vi "Motor Controller.vi"(6 "error in (no error)":errorcluster, 9 "Message Queues in":T1) -> (0 "error out":errorcluster)   [LabVIEW 2024]
uses:
  support/Message Queue/All Message Queues.ctl
  support/Message Queue/Message Cluster.ctl
  support/MotorBoolControlsIndicators.ctl
  support/MotorBoolControls.ctl
  support/MotorSpeedControls.ctl
  support/Message Queue/Enqueue Message (Single).vi
  <vilib>/addons/control/pid/pid.llb/PID (DBL).vi
  support/Message Queue/Message Queue.lvlib
  <vilib>/addons/control/pid/NI_PID_pid.lvlib
panel:
  out "Torque Measurement":dbl
  out "Setpoint Torque":dbl
  out "Setpoint Speed 2":dbl
  out "Setpoint Speed 1":dbl
  out "Sync":bool
  out "Async":bool
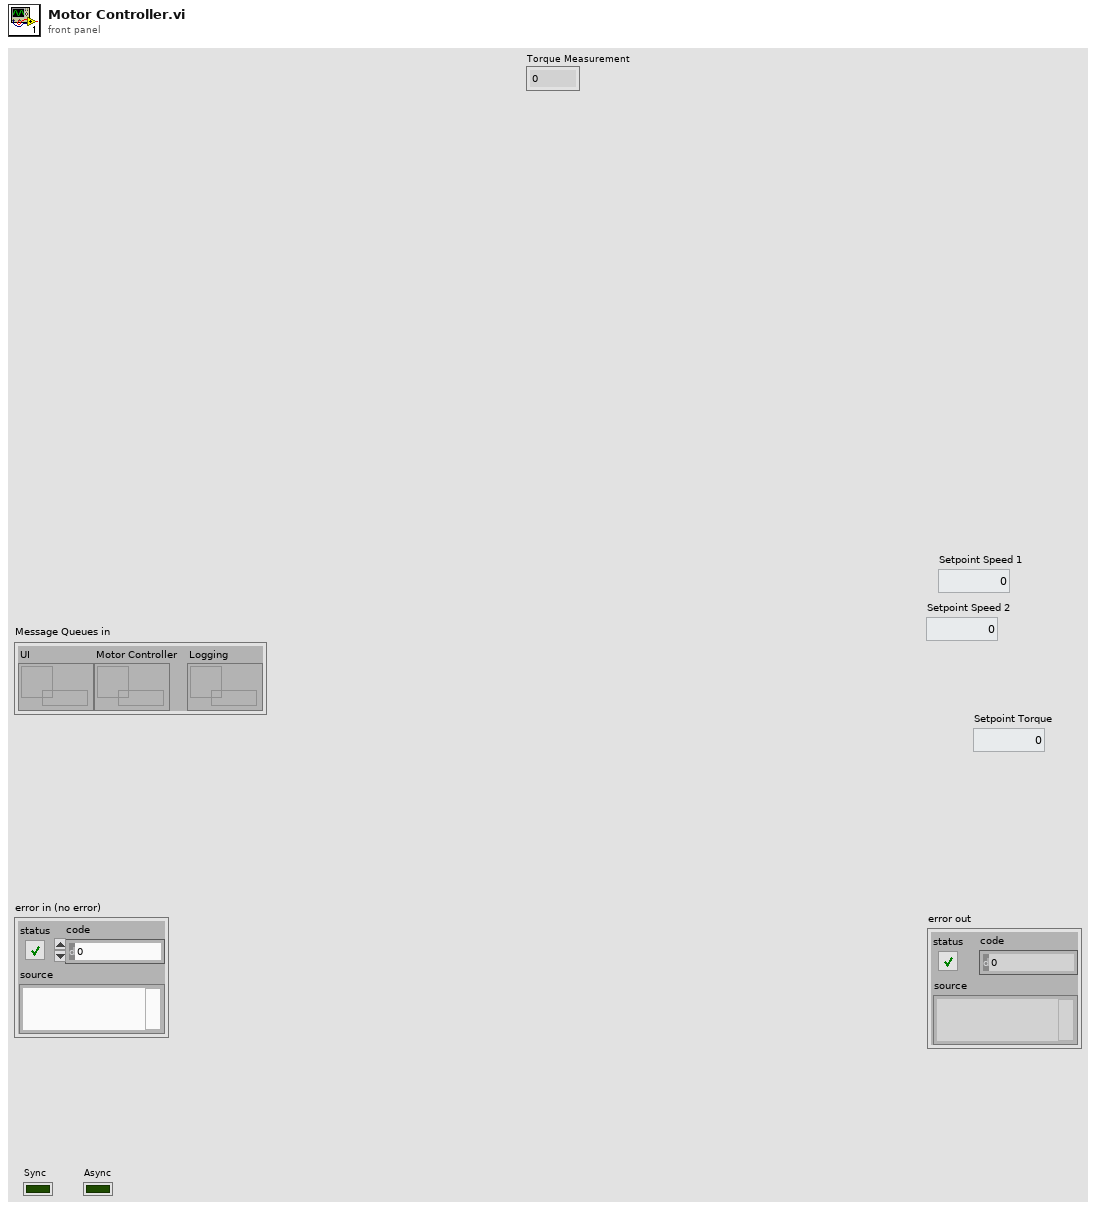
[diagram p1: front panel]
types:
  T1 = typedef "Message Queue.lvlib/All Message Queues.ctl" = cluster{"UI":refnum<queue>, "Motor Controller":refnum<queue>, "Logging":refnum<queue>}
  T2 = typedef "MotorBoolControlsIndicators.ctl" = cluster{"Motor 1 On":bool, "Motor 2 On":bool, "Motors Off":bool, "Start Motor 1 ":bool, "Start Motor 2":bool}
  T3 = typedef "MotorBoolControls.ctl" = cluster{"Motor1On":bool, "Motor2On":bool, "MotorsOff":bool, "StartMotor1":bool, "StartMotor2":bool}
  T4 = typedef "MotorSpeedControls.ctl" = cluster{"SetSpeed1":dbl, "SetSpeed 2":dbl}
  T5 = typedef "MotorStatusIndicators.ctl" = cluster{"Motor 1 Ok":bool, "Motor 2 ok":bool}
  T6 = typedef "ReadSpeed.ctl" = cluster{"SetSpeed1":dbl, "SetSpeed2":dbl, "ReadSpeed1":dbl, "ReadSpeed2":dbl}
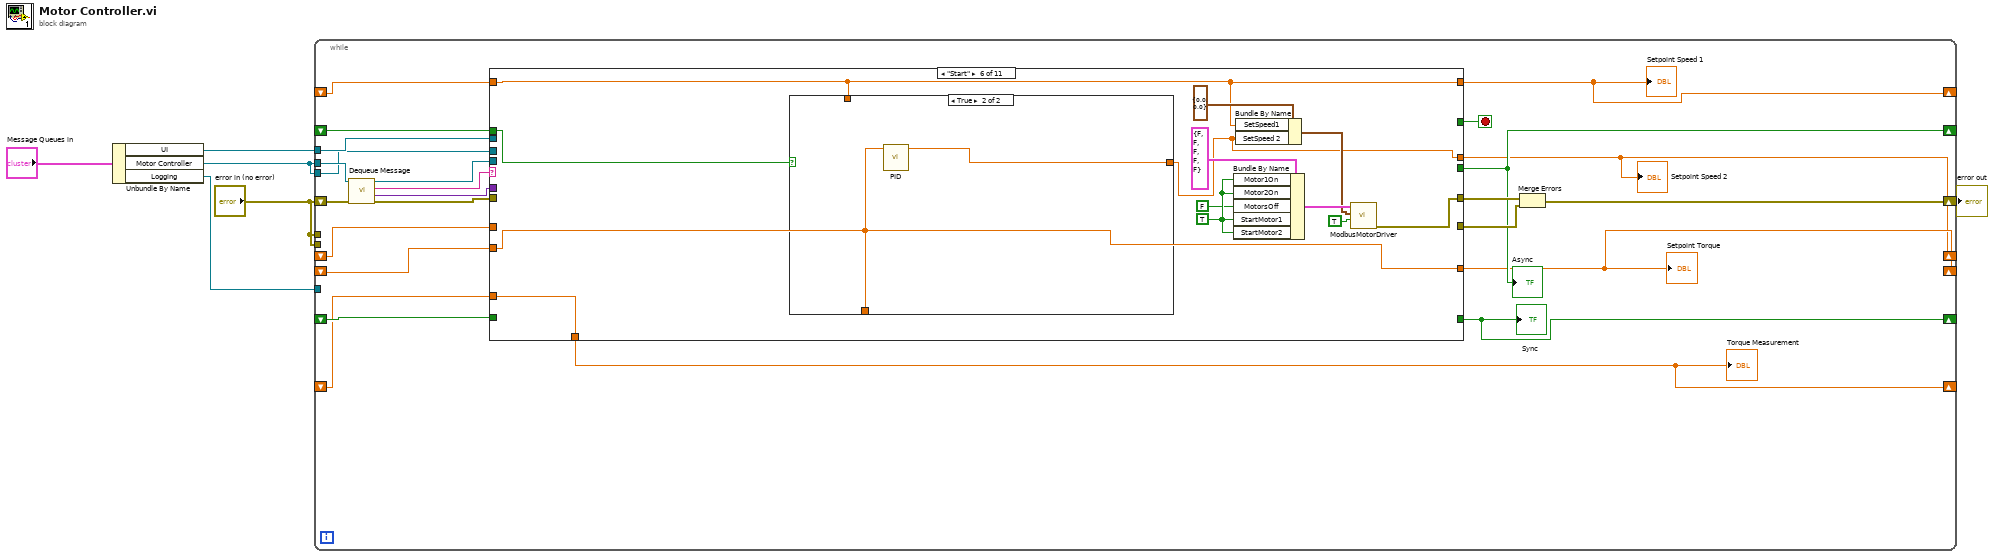
[diagram p0: block diagram]
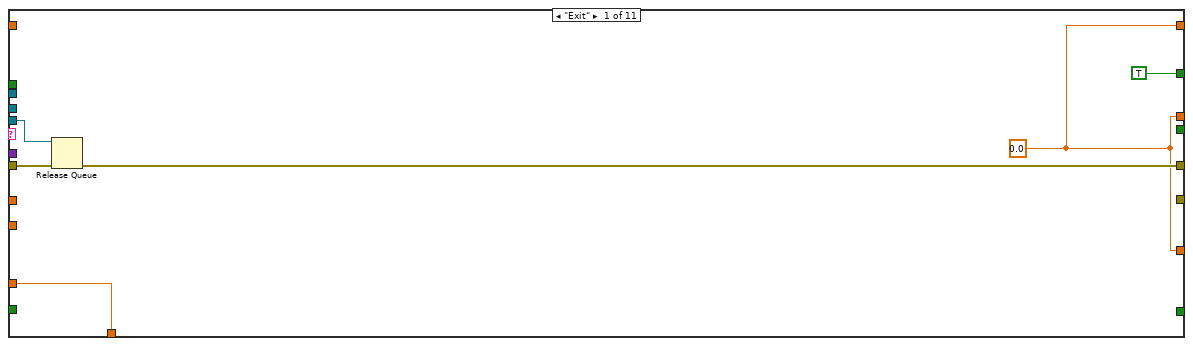
[diagram p2: hidden frame]
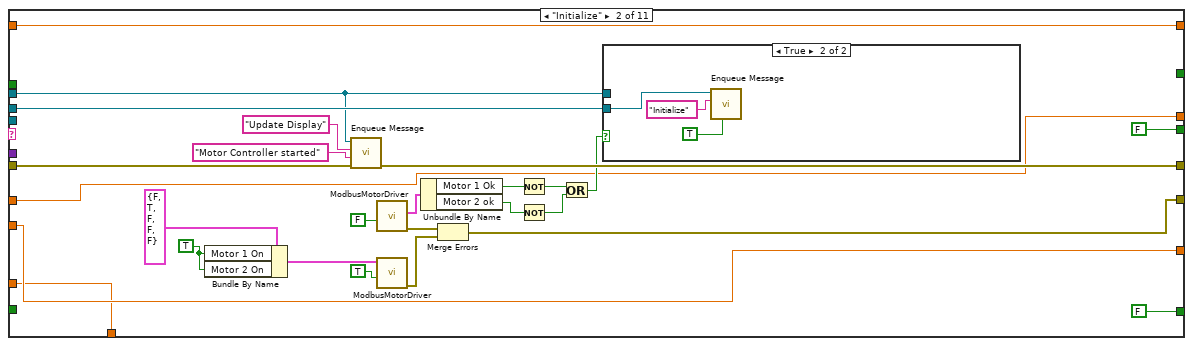
[diagram p3: hidden frame]
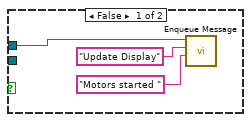
[diagram p4: hidden frame]
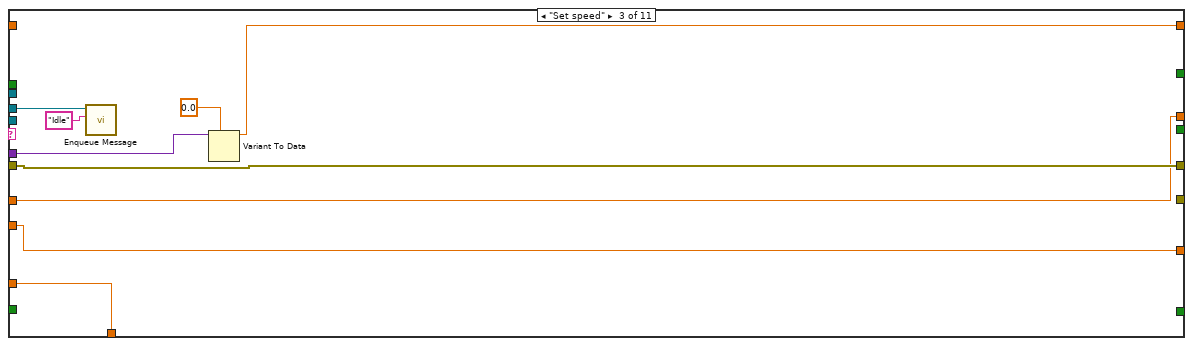
[diagram p5: hidden frame]
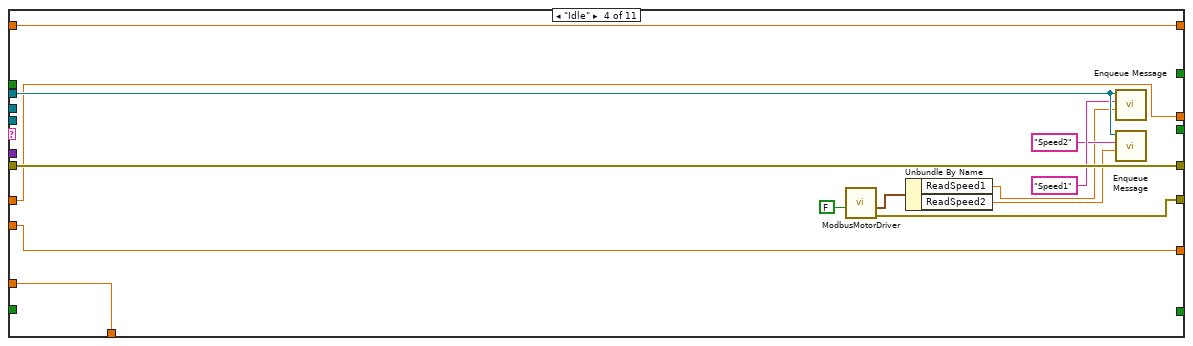
[diagram p6: hidden frame]
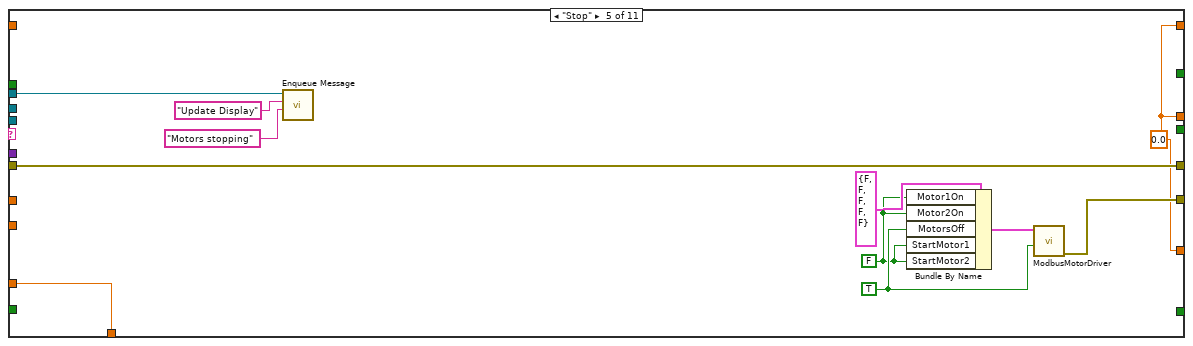
[diagram p7: hidden frame]
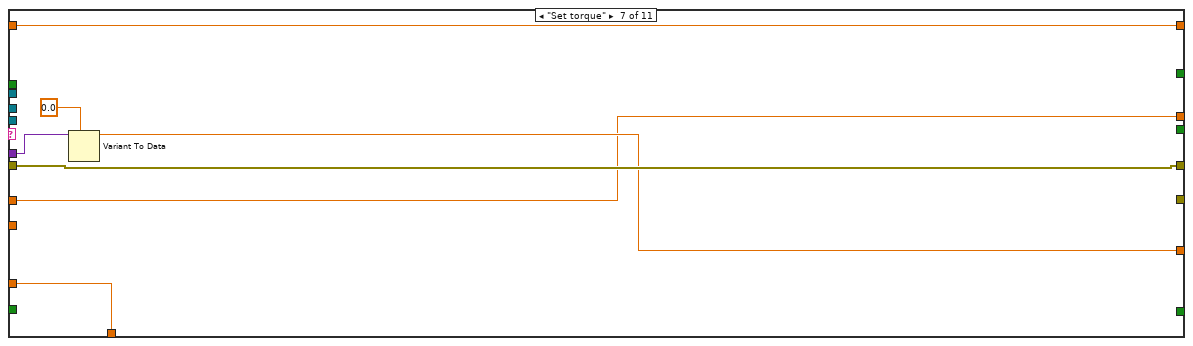
[diagram p9: hidden frame]
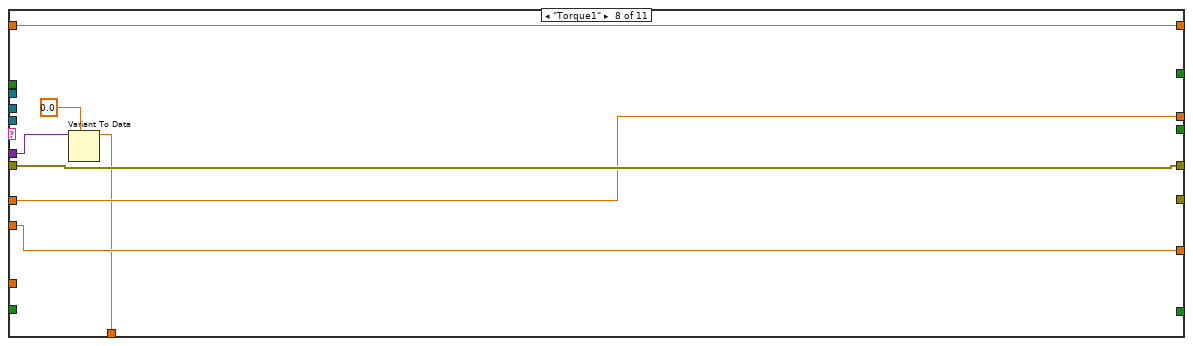
[diagram p10: hidden frame]
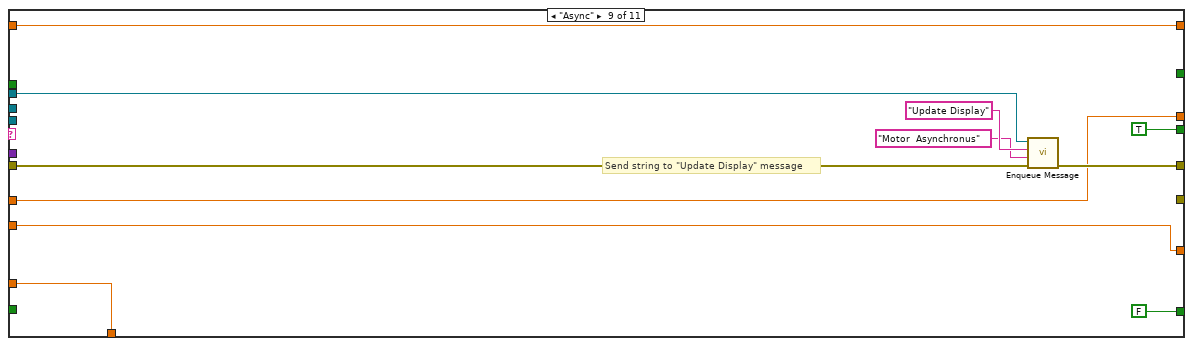
[diagram p11: hidden frame]
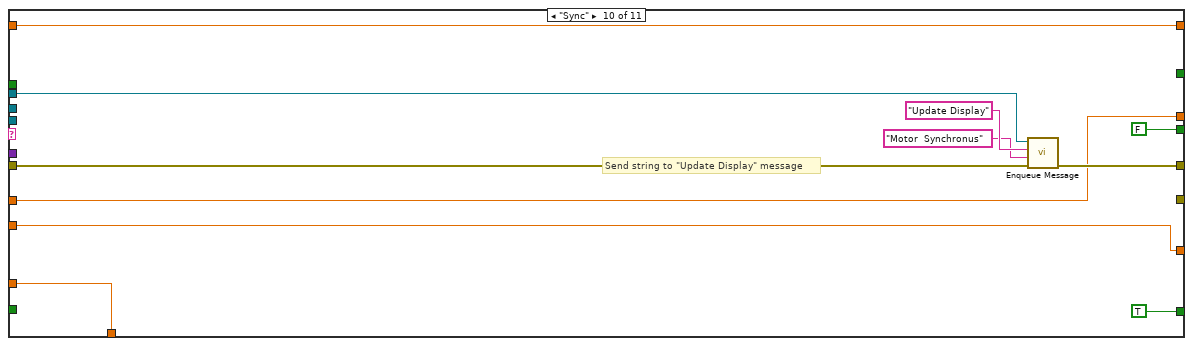
[diagram p12: hidden frame]
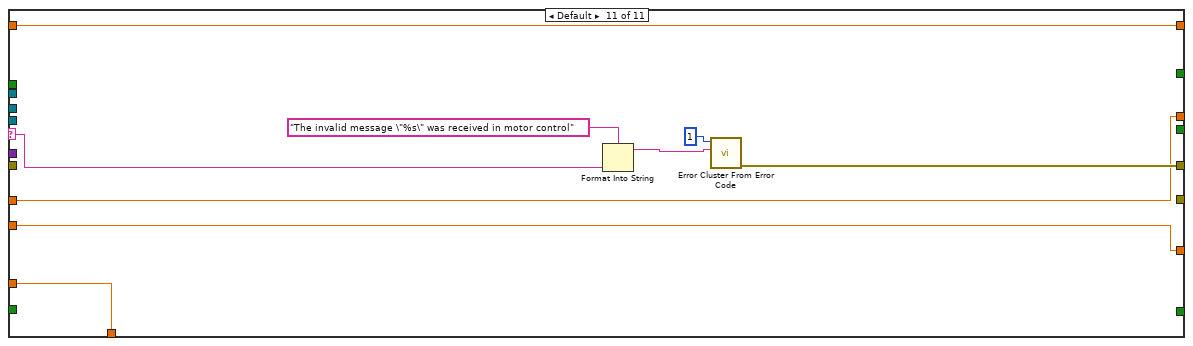
[diagram p13: hidden frame]
diagram:
  n1 = Unbundle By Name("Message Queues in") -> ("UI"=w4:refnum<queue>, "Motor Controller"=w2:refnum<queue>, "Logging"=w3:refnum<queue>)
  n2 = while {
    shift-right: [w19] -> w6
    shift-left: "error in (no error)" -> [w28]
    tunnel: w2 -> [w29]
    tunnel: w4 -> [w24]
    tunnel: w3 -> [_]
    tunnel: "error in (no error)" -> [_]
    tunnel: w2 -> [w22]
    tunnel: "error in (no error)" -> [_]
    shift-right: [w18] -> _
    shift-left: _ -> [w16]
    shift-right: [w17] -> _
    shift-left: _ -> [w15]
    shift-right: [w14] -> _
    shift-left: _ -> [w12]
    shift-right: [w13] -> _
    shift-left: _ -> [w11]
    shift-right: [w10] -> _
    shift-left: _ -> [w9]
    shift-right: [w8] -> _
    shift-left: _ -> [w7]
    stop <- w25 stop-if-true
    n3 = call "Dequeue Message.vi"("error in (no error)"=w28, "Message Queue"=w29) -> ("error out"=w27:errorcluster, "Message Data"=w23:variant, "Message"=w30:string, "dup Message Queue"=w26:refnum<queue>)  [unwired: 6 in]
    n4 = case shown="\"Start\"" w30 {
      selector: w30 -> [_ _ _ _ _ _ _ _ _ _ w158]
      tunnel: [w35 w61 w77 w90 w101 w109 w124 w131 w138 w149 w160] -> w20
      tunnel: w27 -> [w36 w62 w77 w90 w101 _ w124 w131 w139 w150 _]
      tunnel: w26 -> [w33 _ _ _ _ _ _ _ _ _ _]
      tunnel: [TRUE _ _ _ _ _ _ _ _ _ _] -> w25
      tunnel: w24 -> [_ w54 _ w89 w100 _ _ _ w140 w151 _]
      tunnel: w23 -> [_ _ w75 _ _ _ w122 w129 _ _ _]
      tunnel: w22 -> [_ w55 w74 _ _ _ _ _ _ _ _]
      tunnel: [_ FALSE _ _ _ _ _ _ TRUE FALSE _] -> w18
      tunnel: [_ FALSE _ _ _ _ _ _ FALSE TRUE _] -> w17
      tunnel: [_ w46 _ w83 w97 _ _ _ _ _ _] -> w21
      tunnel: w16 -> [_ _ _ _ _ w106 _ _ _ _ _]
      tunnel: w15 -> [_ _ _ _ _ _ _ _ _ _ _]
      tunnel: [w32 w40 w72 w81 w92 w105 w120 w128 w135 w146 w157] -> w14
      tunnel: [w32 w38 w70 w79 w92 w103 w121 w126 w134 w145 w156] -> w13
      tunnel: w12 -> [_ w40 _ w81 _ w105 w120 w128 w135 w146 w157]
      tunnel: w11 -> [_ w38 w70 w79 _ w103 _ w126 w134 w145 w156]
      tunnel: [w32 w39 w71 w80 w92 w104 w119 w127 w133 w144 w155] -> w10
      tunnel: w9 -> [_ w39 w71 w80 _ _ w119 w127 w133 w144 w155]
      tunnel: [w31 w37 w69 w78 w91 w102 w118 w125 w132 w143 w154] -> w8
      tunnel: w7 -> [w31 w37 w69 w78 w91 w102 w118 _ w132 w143 w154]
      frame "Exit" {
        w32 = 0.0
        n5 = Release Queue(queue=w33, error in (no error)=w36) -> (error out=w35:errorcluster)  [unwired: 1 in, 2 out]
      }
      frame "Initialize" {
        w51 = TRUE ("Motor 1 On")
        n6 = Bundle By Name(cluster=T2 {"Motor 1 On"=FALSE, "Motor 2 On"=TRUE, "Motors Off"=FALSE, "Start Motor 1 "=FALSE, "Start Motor 2"=FALSE} ("Motor Bool Control Indicators"), "Motor 1 On"=w51, "Motor 2 On"=w51) -> (w53:T2)
        n7 = call-poly "Enqueue Message.vi"("error in (no error)"=w62, "Message Data"="Motor Controller started", "Message"="Update Display", "Message Queue"=w54) -> ("error out"=w61:errorcluster)  [unwired: 6 in, 1 out]
        n8 = call "ModbusMotorDriver.vi"("Mode"=FALSE) -> ("error IO"=w48:errorcluster, "Motor Status Indicators"=w49:T5)  [unwired: 6 in, 3 out]
        n9 = call "ModbusMotorDriver.vi"("Mode"=TRUE, "Motor Bool Control"=w53) -> ("error IO"=w47:errorcluster)  [unwired: 5 in, 4 out]
        n10 = Unbundle By Name(w49) -> ("Motor 1 Ok"=w43:bool, "Motor 2 ok"=w41:bool)
        n11 = Merge Errors(w48, w47) -> (w46:errorcluster)
        n12 = Not(x=w43) -> (.not. x?=w44:bool)
        n13 = Not(x=w41) -> (.not. x?=w42:bool)
        n14 = Or(x=w44, y=w42) -> (x .or. y?=w56:bool)
        n15 = case shown="True" w56 {
          tunnel: w55 -> [_ w68]
          tunnel: w54 -> [w63 _]
          frame False {
            n16 = call-poly "Enqueue Message.vi"("Message Data"="Motors started ", "Message"="Update Display", "Message Queue"=w63) -> ()  [unwired: 7 in, 2 out]
          }
          frame True {
            n17 = call-poly "Enqueue Message.vi"("Priority Message? (F)"=TRUE, "Message"="Initialize", "Message Queue"=w68) -> ()  [unwired: 7 in, 2 out]
          }
        }
      }
      frame "Set speed" {
        n18 = call-poly "Enqueue Message.vi"("Message"="Idle", "Message Queue"=w74) -> ()  [unwired: 8 in, 2 out]
        n19 = Variant To Data(type=0.0, Variant=w75) -> (data=w72:dbl)  [unwired: 1 in, 1 out]
      }
      frame "Idle" {
        n20 = call "ModbusMotorDriver.vi"("Mode"=FALSE) -> ("error IO"=w83:errorcluster, "Read Speed"=w86:T6)  [unwired: 6 in, 3 out]
        n21 = Unbundle By Name(w86) -> ("ReadSpeed1"=w85:dbl, "ReadSpeed2"=w84:dbl)
        n22 = call-poly "Enqueue Message.vi"("Message Data"=w85, "Message"="Speed1", "Message Queue"=w89) -> ()  [unwired: 7 in, 2 out]
        n23 = call-poly "Enqueue Message.vi"("Message Data"=w84, "Message"="Speed2", "Message Queue"=w89) -> ()  [unwired: 7 in, 2 out]
      }
      frame "Stop" {
        w92 = 0.0
        w93 = FALSE ("Motor1On")
        w95 = TRUE ("stop")
        n24 = call-poly "Enqueue Message.vi"("Message Data"="Motors stopping" ("Message"), "Message"="Update Display", "Message Queue"=w100) -> ()  [unwired: 7 in, 2 out]
        n25 = Bundle By Name(cluster=T3 {"Motor1On"=FALSE, "Motor2On"=FALSE, "MotorsOff"=FALSE, "StartMotor1"=FALSE, "StartMotor2"=FALSE} ("Motor Bool Control"), "Motor1On"=w93, "Motor2On"=w93, "MotorsOff"=w95, "StartMotor1"=w93, "StartMotor2"=w93) -> (w94:T3)
        n26 = call "ModbusMotorDriver.vi"("Mode"=w95, "Motor Bool Control"=w94) -> ("error IO"=w97:errorcluster)  [unwired: 5 in, 4 out]
      }
      frame "Start" {
        w111 = TRUE
        n27 = case shown="True" w106 {
          tunnel: [w115 w116] -> w104
          tunnel: w105 -> [w115 _]
          tunnel: w103 -> [_ w117]
          frame False {
          }
          frame True {
            n28 = call-poly <vilib>:"PID.vi"("setpoint"=w117) -> ("output"=w116:dbl)  [unwired: 9 in, 1 out]
          }
        }
        n29 = Bundle By Name(cluster=T3 {"Motor1On"=FALSE, "Motor2On"=FALSE, "MotorsOff"=FALSE, "StartMotor1"=FALSE, "StartMotor2"=FALSE} ("Motor Bool Control"), "Motor1On"=w111, "Motor2On"=w111, "MotorsOff"=FALSE, "StartMotor1"=w111, "StartMotor2"=w111) -> (w112:T3)
        n30 = Bundle By Name(cluster=T4 {"SetSpeed1"=0.0, "SetSpeed 2"=0.0} ("M;otor Speed Controls"), "SetSpeed1"=w105, "SetSpeed 2"=w104) -> (w107:T4)
        n31 = call "ModbusMotorDriver.vi"("Mode"=TRUE, "M;otor Speed Controls"=w107, "Motor Bool Control"=w112) -> ("error IO"=w109:errorcluster)  [unwired: 4 in, 4 out]
      }
      frame "Set torque" {
        n32 = Variant To Data(type=0.0, Variant=w122) -> (data=w121:dbl)  [unwired: 1 in, 1 out]
      }
      frame "Torque1" {
        n33 = Variant To Data(type=0.0, Variant=w129) -> (data=w125:dbl)  [unwired: 1 in, 1 out]
      }
      frame "Async" {
        # "Send string to \"Update Display\" message"
        n34 = call-poly "Enqueue Message.vi"("error in (no error)"=w139, "Message Data"="Motor  Asynchronus" ("\"Do Something\" button pressed"), "Message"="Update Display", "Message Queue"=w140) -> ("error out"=w138:errorcluster)  [unwired: 6 in, 1 out]
      }
      frame "Sync" {
        # "Send string to \"Update Display\" message"
        n35 = call-poly "Enqueue Message.vi"("error in (no error)"=w150, "Message Data"="Motor  Synchronus" ("\"Do Something\" button pressed"), "Message"="Update Display", "Message Queue"=w151) -> ("error out"=w149:errorcluster)  [unwired: 6 in, 1 out]
      }
      frame Default {
        n36 = Format Into String(format string="The invalid message \"%s\" was received in motor control", w158) -> (resulting string=w161:string)  [unwired: 2 in, 1 out]
        n37 = call <vilib>:"Error Cluster From Error Code.vi"("error message (\"\")"=w161, "error code (0)"=1) -> ("error out"=w160:errorcluster)  [unwired: 7 in]
      }
    }
    "Async" <- w18
    "Sync" <- w17
    "Setpoint Speed 1" <- w14
    "Setpoint Speed 2" <- w10
    "Setpoint Torque" <- w13
    "Torque Measurement" <- w8
    n38 = Merge Errors(w20, w21) -> (w19:errorcluster)
  }
  "error out" <- w6
